vi "x!.vi"(1 "x":i32) -> (0 "x!":i32)   [LabVIEW 2009]
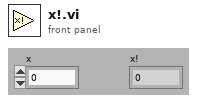
[diagram p1: front panel]
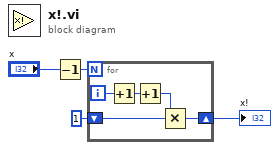
[diagram p0: block diagram]
diagram:
  n1 = Decrement(x="x") -> (x-1=w1:i32)
  n2 = for {
    N: w1 -> [_]
    shift-right: [w9] -> w4
    shift-left: 1 ("y") -> [w8]
    i -> [w7]
    n3 = Increment(x=w7) -> (x+1=w6:i32)
    n4 = Increment(x=w6) -> (x+1=w5:i32)
    n5 = Multiply(x=w5, y=w8) -> (x*y=w9:i32)
  }
  "x!" <- w4
